vi "main_new.vi"() -> ()   [LabVIEW 2019]
uses:
  Controls/data.ctl
  Estats.ctl
panel:
  out "Pict Ring":u16(ring)
  in  "Prova":bool
  out "Diners":string
  in  "Stop Button":bool
  out "Diàleg":string
  out "Canvi":string
  in  "Orange":bool
  in  "Lemond":bool
  in  "Apple":bool
  in  "50cents":bool
  in  "20cents":bool
  in  "10cents":bool
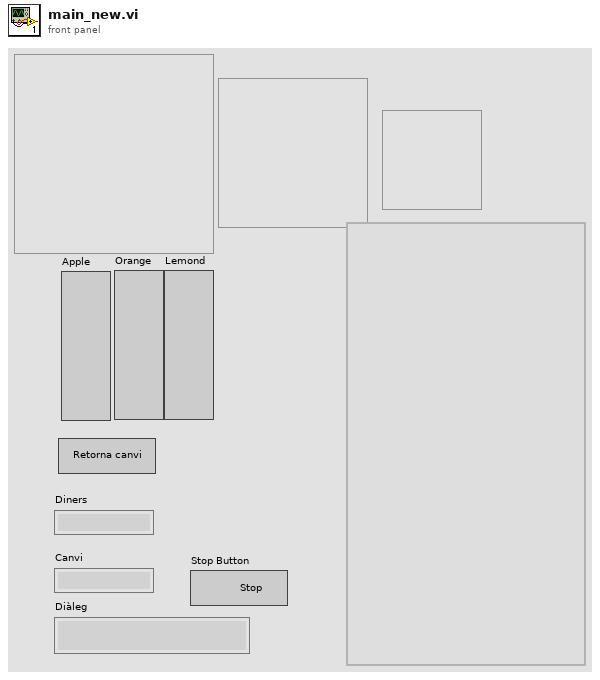
[diagram p1: front panel]
types:
  T1 = typedef "Estats.ctl" = enum16{"Init", "Wait for Event", "Exit", "Return Money", "Lemond", "Apple", "Orange", "Deliver", "50cents", "20cents", "10cents"}
  T2 = typedef "data.ctl" = cluster{"Diners":dbl, "Han triat veguda":bool}
  T3 = enum8{"Enabled", "Disabled", "Disabled and Grayed Out"}
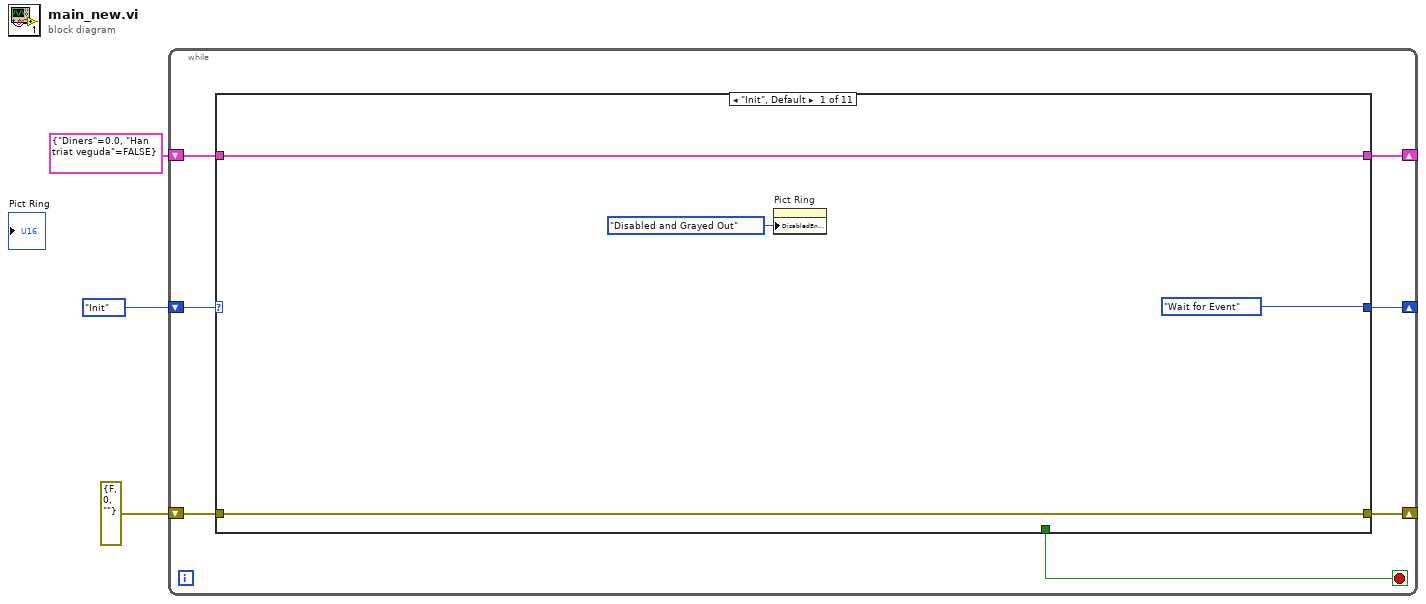
[diagram p0: block diagram]
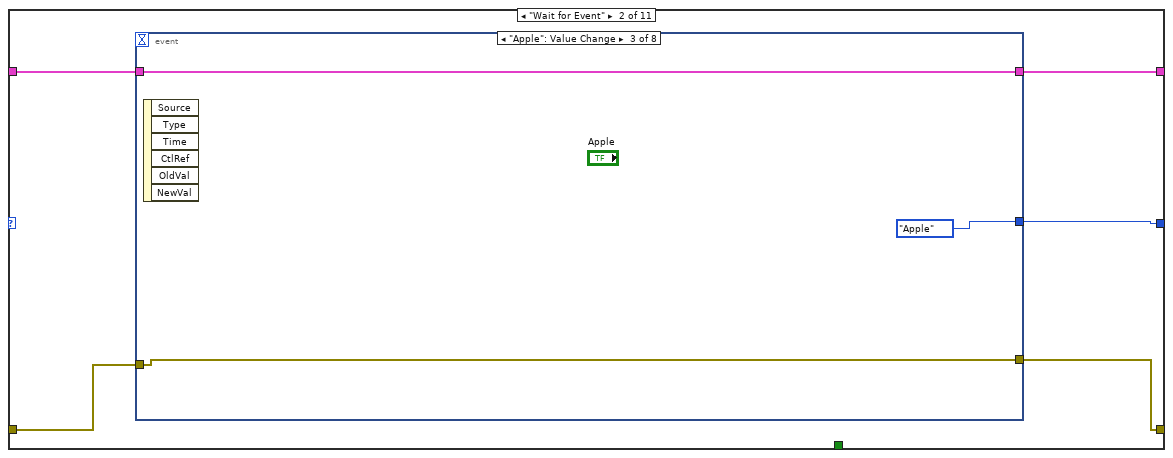
[diagram p2: hidden frame]
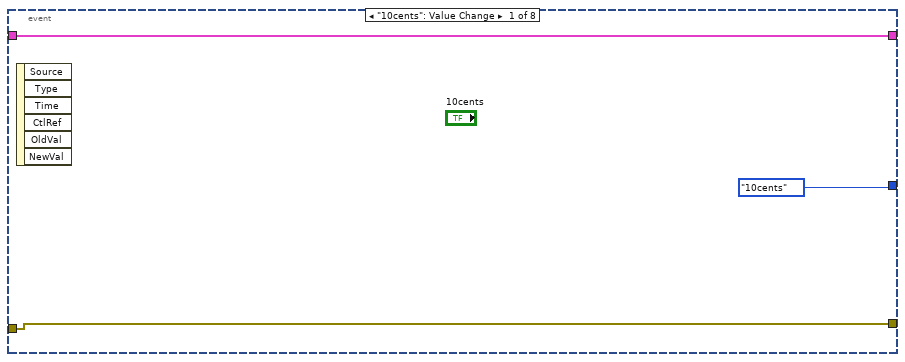
[diagram p3: hidden frame]
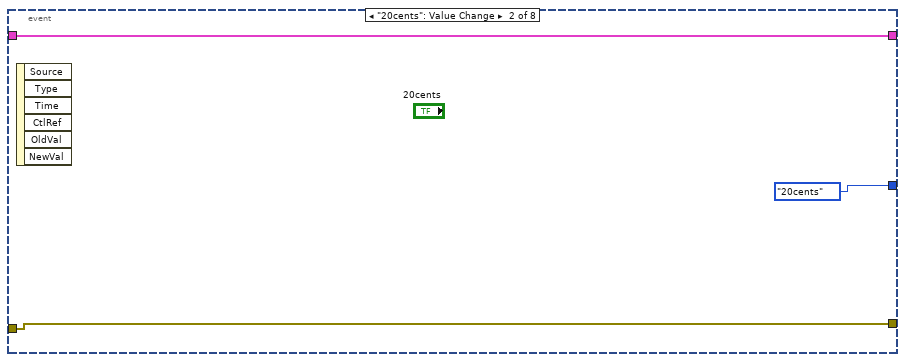
[diagram p4: hidden frame]
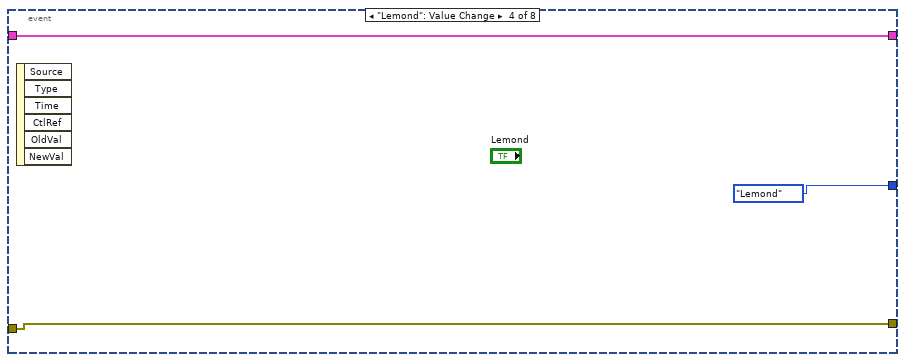
[diagram p5: hidden frame]
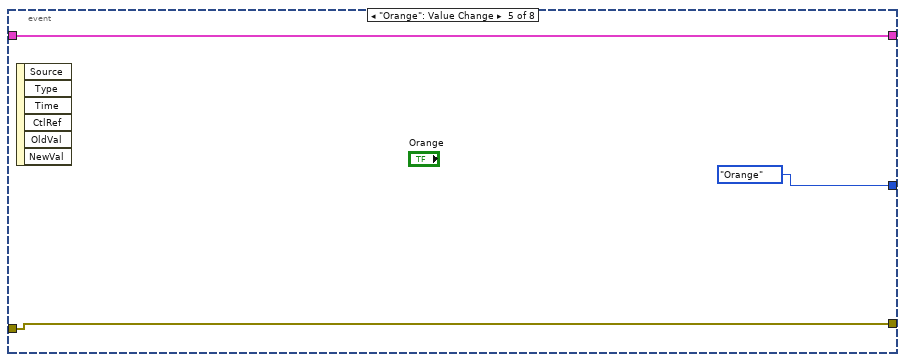
[diagram p6: hidden frame]
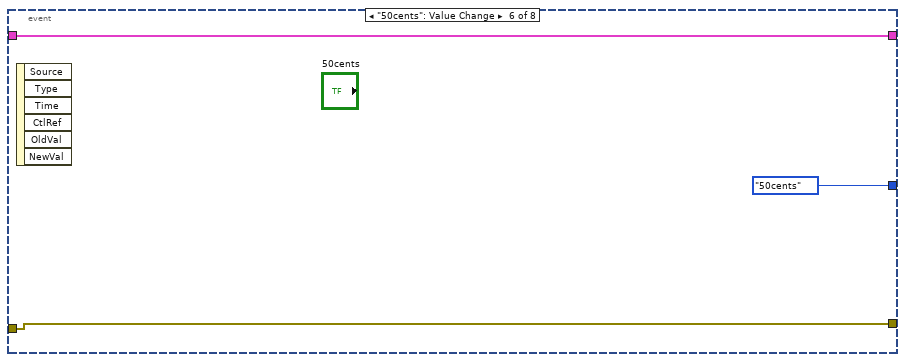
[diagram p7: hidden frame]
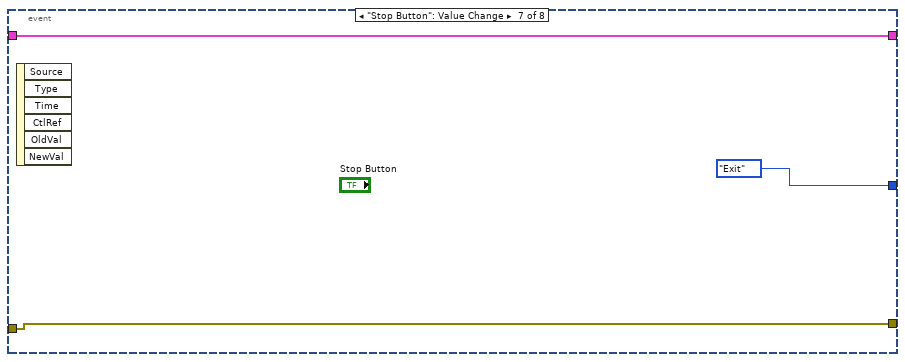
[diagram p8: hidden frame]
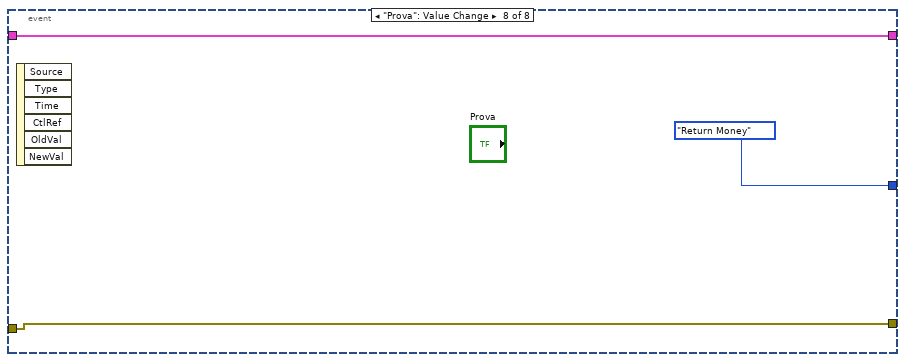
[diagram p9: hidden frame]
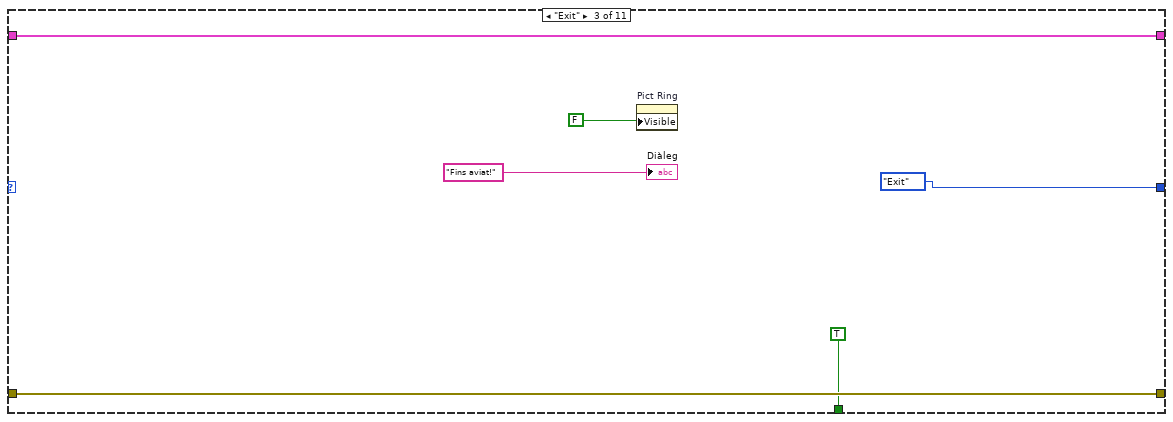
[diagram p10: hidden frame]
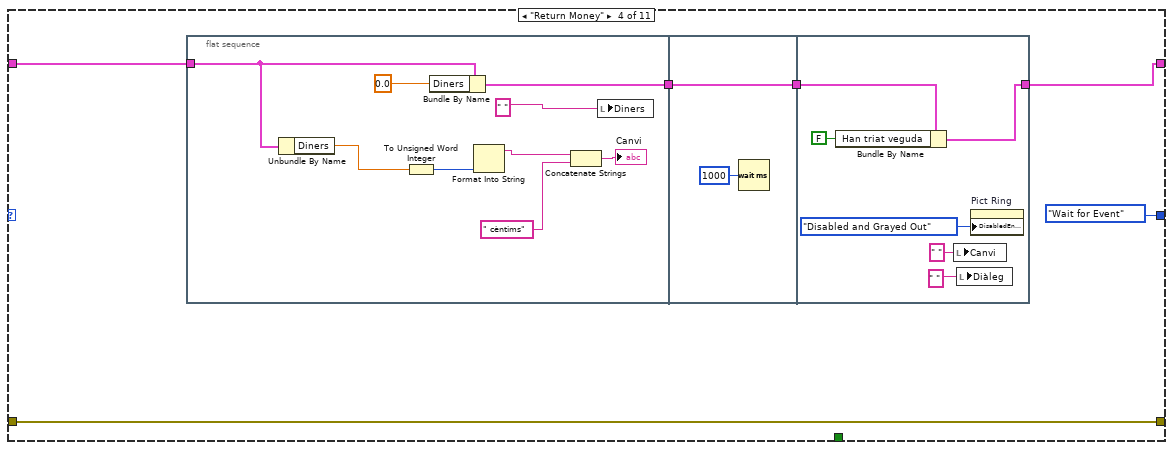
[diagram p11: hidden frame]
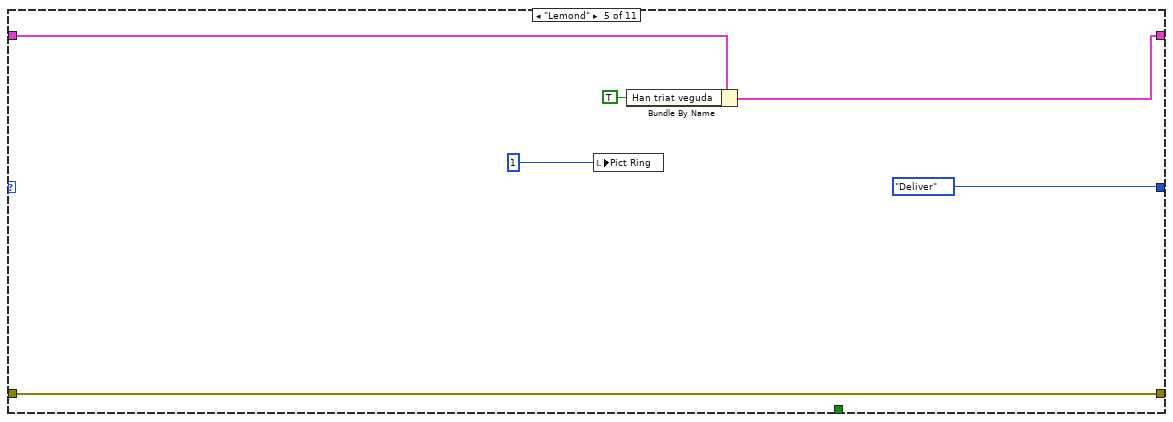
[diagram p12: hidden frame]
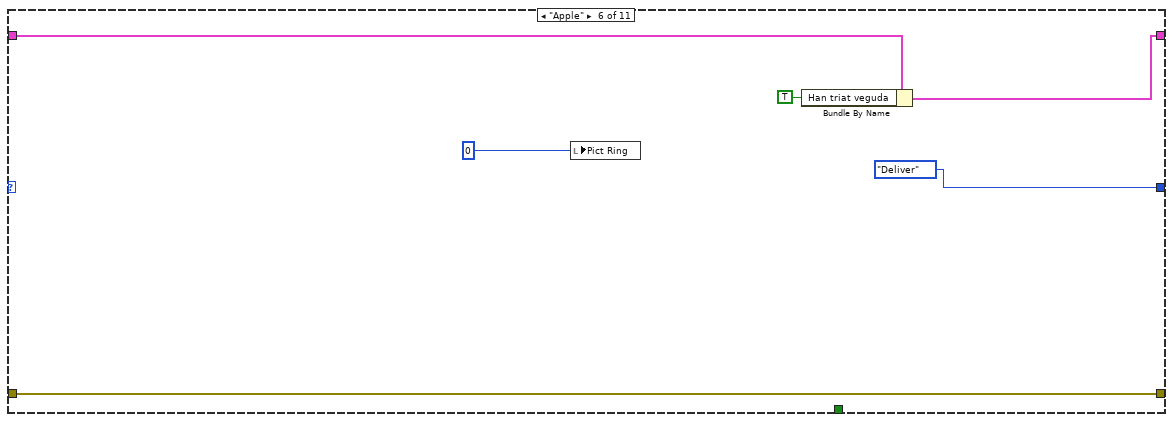
[diagram p13: hidden frame]
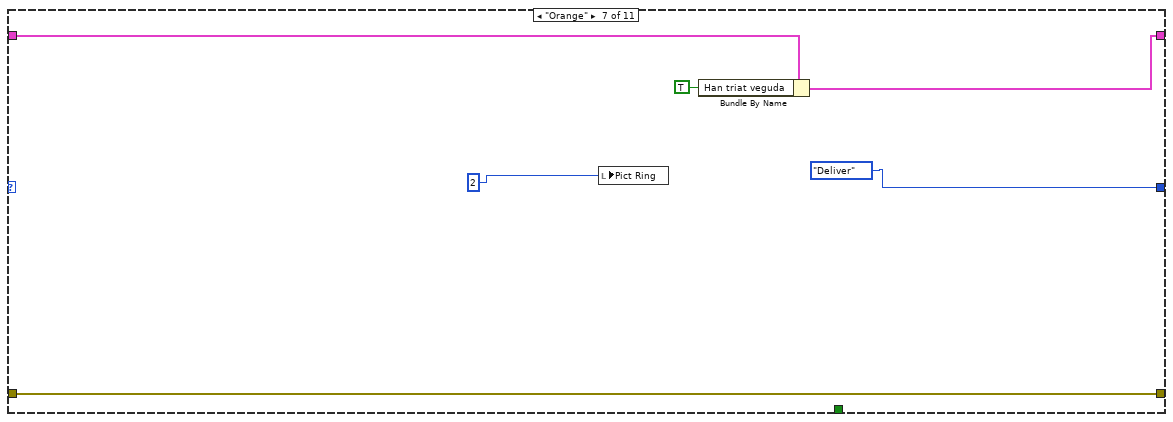
[diagram p14: hidden frame]
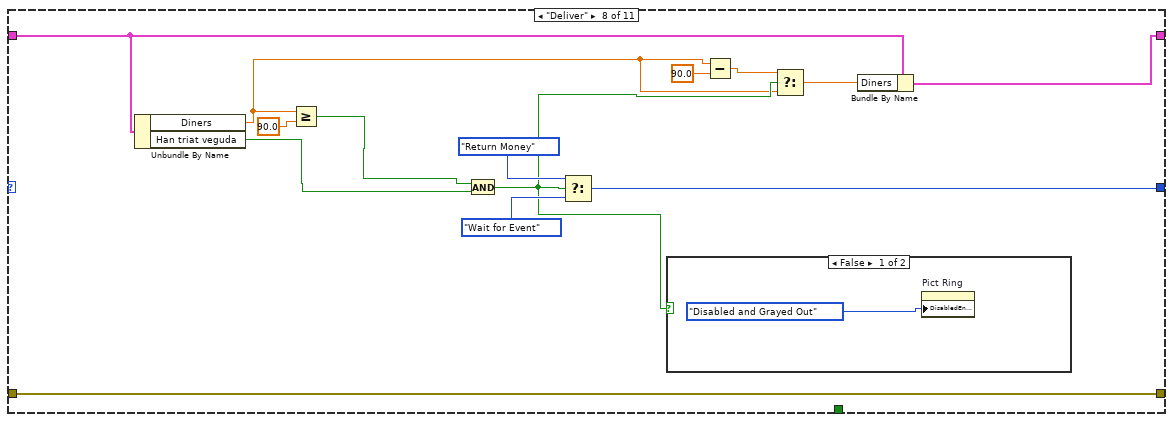
[diagram p15: hidden frame]
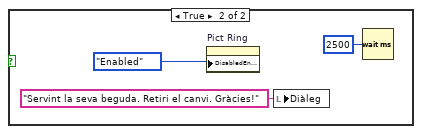
[diagram p16: hidden frame]
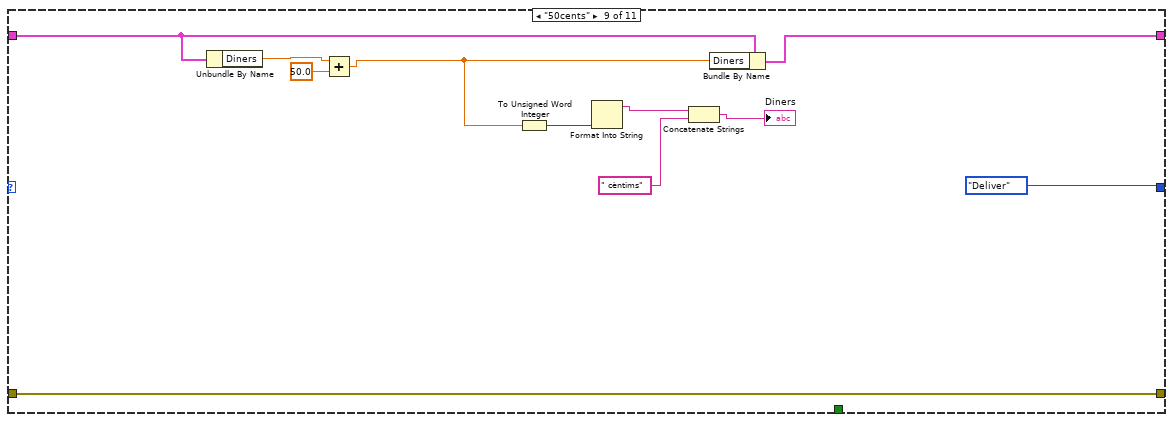
[diagram p17: hidden frame]
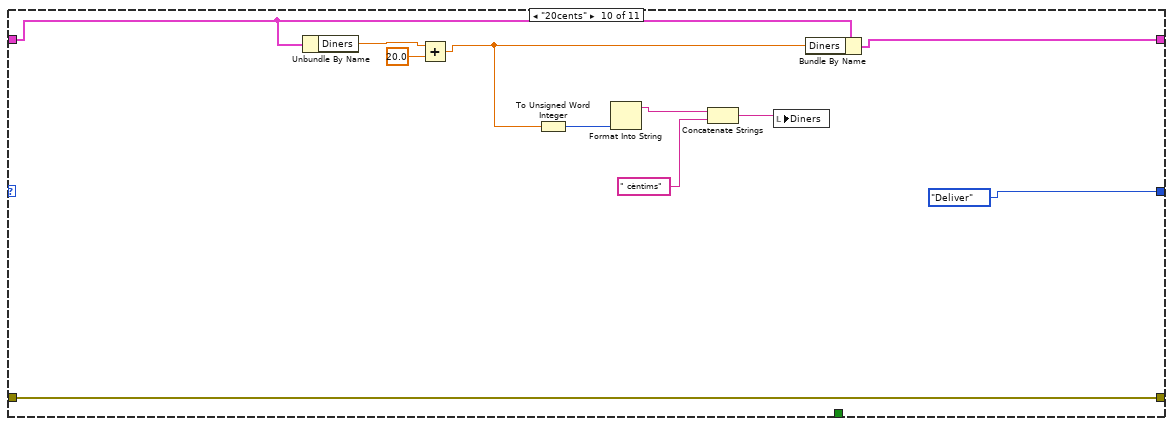
[diagram p18: hidden frame]
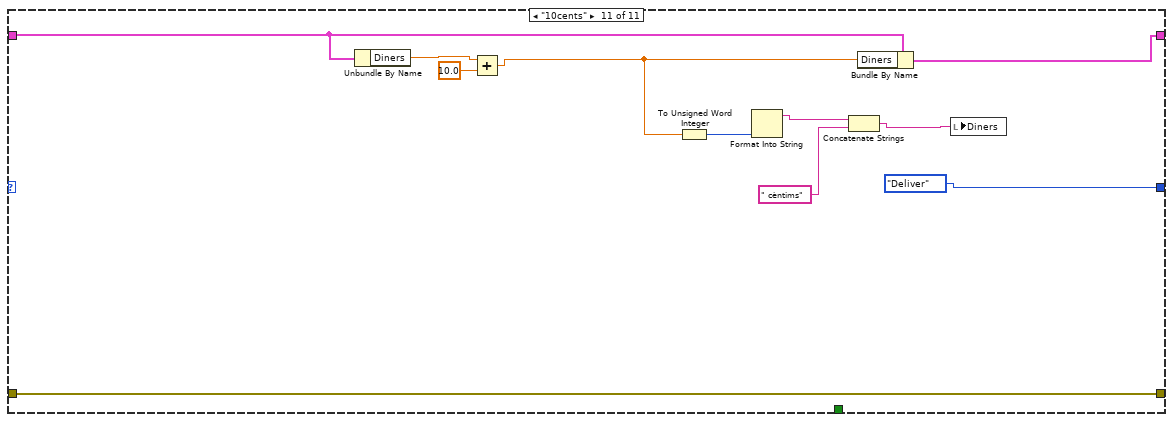
[diagram p19: hidden frame]
diagram:
  n1 = while {
    shift-right: [w5] -> _
    shift-left: Estats."Init" ("Enum") -> [w10]
    shift-right: [w6] -> _
    shift-left: T2 {"Diners"=0.0, "Han triat veguda"=FALSE} ("Cluster") -> [w9]
    shift-right: [w7] -> _
    shift-left: errorcluster {"status"=FALSE, "code"=0, "source"=""} ("error constant") -> [w8]
    stop <- w4 stop-if-true
    n2 = case shown="\"Init\", Default" w10 {
      tunnel: w9 -> [w14 w18 w48 w53 w76 w81 w87 w98 w115 w126 w137]
      tunnel: w8 -> [w12 w17 w47 w54 w77 w83 w89 w101 w118 w129 w140]
      tunnel: [w12 w16 w47 w54 w77 w83 w89 w101 w118 w129 w140] -> w7
      tunnel: [w14 w19 w48 w52 w75 w80 w86 w97 w114 w125 w136] -> w6
      tunnel: [Estats."Wait for Event" ("Enum") w15 Estats."Exit" ("Enum") Estats."Wait for Event" ("Enum") Estats."Deliver" ("Enum") Estats."Deliver" ("Enum") Estats."Deliver" ("Enum") w102 Estats."Deliver" ("Enum") Estats."Deliver" ("Enum") Estats."Deliver" ("Enum")] -> w5
      tunnel: [_ _ TRUE ("stop") _ _ _ _ _ _ _ _] -> w4
      frame "Init", Default {
        n3 = property on="Pict Ring" class="Ring (strict)"("DisabledEnum"=T3."Disabled and Grayed Out" ("Disabled")) -> ()  [unwired: 2 in, 2 out]
      }
      frame "Wait for Event" {
        n4 = event shown="[2] \"Apple\": Value Change" {
          selector: _ -> [_ _ _ _ _ _ _ _]
          dyn-events: _ -> [_ _ _ _ _ _ _ _]
          timeout: _ -> [_ _ _ _ _ _ _ _]
          tunnel: [w21 w24 w26 w29 w32 w35 w38 w41] -> w19
          tunnel: w18 -> [w21 w24 w26 w29 w32 w35 w38 w41]
          tunnel: w17 -> [w20 w23 w27 w30 w33 w36 w39 w42]
          tunnel: [w20 w23 w27 w30 w33 w36 w39 w42] -> w16
          tunnel: [Estats."10cents" ("Enum") Estats."20cents" ("Enum") Estats."Apple" ("Enum") Estats."Lemond" ("Enum") Estats."Orange" ("Enum") Estats."50cents" ("Enum") Estats."Exit" ("Enum") Estats."Return Money" ("Enum")] -> w15
          event "10cents": Value Change {
            n5 = event-data() -> ()  [unwired: 1 in, 6 out]
          }
          event "20cents": Value Change {
            n6 = event-data() -> ()  [unwired: 1 in, 6 out]
          }
          event "Apple": Value Change {
            n7 = event-data() -> ()  [unwired: 1 in, 6 out]
          }
          event "Lemond": Value Change {
            n8 = event-data() -> ()  [unwired: 1 in, 6 out]
          }
          event "Orange": Value Change {
            n9 = event-data() -> ()  [unwired: 1 in, 6 out]
          }
          event "50cents": Value Change {
            n10 = event-data() -> ()  [unwired: 1 in, 6 out]
          }
          event "Stop Button": Value Change {
            n11 = event-data() -> ()  [unwired: 1 in, 6 out]
          }
          event "Prova": Value Change {
            n12 = event-data() -> ()  [unwired: 1 in, 6 out]
          }
        }
      }
      frame "Exit" {
        n13 = property on="Pict Ring" class="Ring (strict)"("Visible"=FALSE) -> ()  [unwired: 2 in, 2 out]
        "Diàleg" <- "Fins aviat!" ("Estat")
      }
      frame "Return Money" {
        n14 = flat-sequence {
          tunnel: w53 -> [w62]
          tunnel: [w61] -> w51
          tunnel: w51 -> [w66]
          tunnel: [w66] -> w50
          tunnel: [w70] -> w52
          tunnel: w50 -> [w68]
          frame #0 {
            n15 = Unbundle By Name(w62) -> ("Diners"=w59:dbl)
            n16 = To Unsigned Word Integer(number=w59) -> (unsigned 16bit integer=w60:u16)
            n17 = Bundle By Name(cluster=w62, "Diners"=0.0) -> (w61:T2)
            n18 = Format Into String(w60) -> (resulting string=w63:string)  [unwired: 3 in, 1 out]
            n19 = Concatenate Strings(w63, " cèntims" ("string")) -> (→"Canvi":string)
            n20 = local write "Diners"(" " ("Canvi")) -> ()
          }
          frame #1 {
            n21 = Wait (ms)(milliseconds to wait=u32 1000) -> ()  [unwired: 1 out]
          }
          frame #2 {
            n22 = Bundle By Name(cluster=w68, "Han triat veguda"=FALSE) -> (w70:T2)
            n23 = local write "Canvi"(" " ("Canvi")) -> ()
            n24 = local write "Diàleg"(" " ("Canvi")) -> ()
            n25 = property on="Pict Ring" class="Ring (strict)"("DisabledEnum"=T3."Disabled and Grayed Out" ("Disabled")) -> ()  [unwired: 2 in, 2 out]
          }
        }
      }
      frame "Lemond" {
        n26 = local write "Pict Ring"(u16 1 ("Ring")) -> ()
        n27 = Bundle By Name(cluster=w76, "Han triat veguda"=TRUE) -> (w75:T2)
      }
      frame "Apple" {
        n28 = local write "Pict Ring"(u16 0 ("Ring")) -> ()
        n29 = Bundle By Name(cluster=w81, "Han triat veguda"=TRUE) -> (w80:T2)
      }
      frame "Orange" {
        n30 = local write "Pict Ring"(u16 2 ("Ring")) -> ()
        n31 = Bundle By Name(cluster=w87, "Han triat veguda"=TRUE) -> (w86:T2)
      }
      frame "Deliver" {
        n32 = Unbundle By Name(w98) -> ("Diners"=w91:dbl, "Han triat veguda"=w100:bool)
        n33 = Greater Or Equal?(x=w91, y=90.0 ("x")) -> (x >= y?=w99:bool)
        n34 = And(x=w99, y=w100) -> (x .and. y?=w93:bool)
        n35 = Select(t=Estats."Return Money" ("Enum"), s=w93, f=Estats."Wait for Event" ("Enum")) -> (s? t:f=w102:T1)
        n36 = case shown="False" w93 {
          frame False {
            n37 = property on="Pict Ring" class="Ring (strict)"("DisabledEnum"=T3."Disabled and Grayed Out" ("Disabled")) -> ()  [unwired: 2 in, 2 out]
          }
          frame True {
            n38 = property on="Pict Ring" class="Ring (strict)"("DisabledEnum"=T3."Enabled" ("Disabled")) -> ()  [unwired: 2 in, 2 out]
            n39 = local write "Diàleg"("Servint la seva beguda. Retiri el canvi. Gràcies!" ("Estat")) -> ()
            n40 = Wait (ms)(milliseconds to wait=u32 2500) -> ()  [unwired: 1 out]
          }
        }
        n41 = Subtract(x=w91, y=90.0) -> (x-y=w95:dbl)
        n42 = Select(t=w95, s=w93, f=w91) -> (s? t:f=w96:dbl)
        n43 = Bundle By Name(cluster=w98, "Diners"=w96) -> (w97:T2)
      }
      frame "50cents" {
        n44 = Unbundle By Name(w115) -> ("Diners"=w116:dbl)
        n45 = Add(x=w116, y=50.0) -> (x+y=w110:dbl)
        n46 = To Unsigned Word Integer(number=w110) -> (unsigned 16bit integer=w111:u16)
        n47 = Format Into String(w111) -> (resulting string=w109:string)  [unwired: 3 in, 1 out]
        n48 = Concatenate Strings(w109, " cèntims" ("string")) -> (→"Diners":string)
        n49 = Bundle By Name(cluster=w115, "Diners"=w110) -> (w114:T2)
      }
      frame "20cents" {
        n50 = Unbundle By Name(w126) -> ("Diners"=w127:dbl)
        n51 = Add(x=w127, y=20.0) -> (x+y=w121:dbl)
        n52 = To Unsigned Word Integer(number=w121) -> (unsigned 16bit integer=w123:u16)
        n53 = Format Into String(w123) -> (resulting string=w122:string)  [unwired: 3 in, 1 out]
        n54 = Concatenate Strings(w122, " cèntims" ("string")) -> (w120:string)
        n55 = local write "Diners"(w120) -> ()
        n56 = Bundle By Name(cluster=w126, "Diners"=w121) -> (w125:T2)
      }
      frame "10cents" {
        n57 = Unbundle By Name(w137) -> ("Diners"=w138:dbl)
        n58 = Add(x=w138, y=10.0) -> (x+y=w132:dbl)
        n59 = To Unsigned Word Integer(number=w132) -> (unsigned 16bit integer=w134:u16)
        n60 = Format Into String(w134) -> (resulting string=w135:string)  [unwired: 3 in, 1 out]
        n61 = Concatenate Strings(w135, " cèntims" ("string")) -> (w131:string)
        n62 = Bundle By Name(cluster=w137, "Diners"=w132) -> (w136:T2)
        n63 = local write "Diners"(w131) -> ()
      }
    }
  }
